vi "Subpanel Connect Event.vi"(8 "error in (no error)":errorcluster, 11 "CIF_UI in":refnum<class "CIF_UI.lvclass">) -> (0 "error out":errorcluster)   [LabVIEW 2021, in "CIF_UI.lvclass"]
uses:
  CIF_UI.lvclass
  CIF_UI.lvclass/CIF_UI.ctl
  Typedef/New Connection Event Data.ctl
  <vilib>/gRPC/LabVIEW gRPC Library/Shared/grpcId.ctl
  <vilib>/gRPC/LabVIEW gRPC Library/grpc-lvsupport-release.lvlib
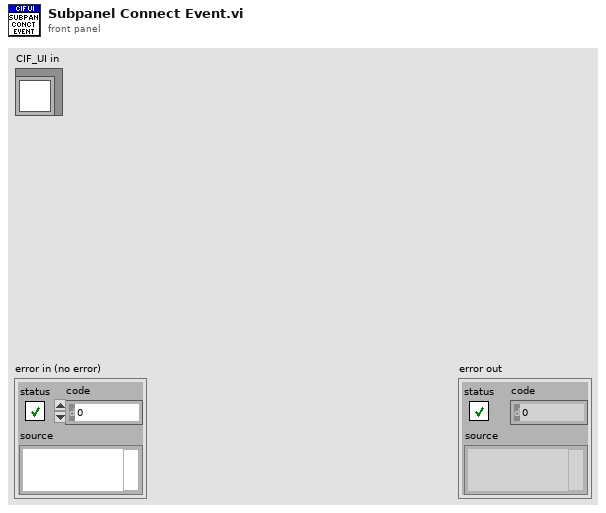
[diagram p1: front panel]
types:
  T1 = typedef "CIF_UI.lvclass/New Connection Event Data.ctl" = cluster{"Manager gRPC ID":T2, "IP Address":string, "Connected":bool}
  T2 = typedef "grpc-lvsupport-release.lvlib/grpcId.ctl" = u64
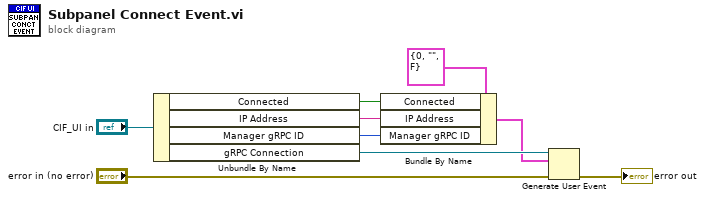
[diagram p0: block diagram]
diagram:
  n1 = Unbundle By Name("CIF_UI in") -> ("Connected"=w2:bool, "IP Address"=w3:string, "Manager gRPC ID"=w4:T2, "gRPC Connection"=w6:refnum<user-event>)
  n2 = Bundle By Name(cluster=T1 {"Manager gRPC ID"=0, "IP Address"="", "Connected"=FALSE} ("event data"), "Connected"=w2, "IP Address"=w3, "Manager gRPC ID"=w4) -> (w1:T1)
  n3 = Generate User Event(user event=w6, event data cluster=w1, error in="error in (no error)") -> (error out=→"error out":errorcluster)  [unwired: 1 in, 1 out]
